vi "Text Description.vi"(11 "Relabel in":refnum<class "AddOuterEnvelope.lvclass">) -> (2 "Description":string, 3 "Relabel out":refnum<class "AddOuterEnvelope.lvclass">)   [LabVIEW 2011, in "Messenging.lvlib" / "AddOuterEnvelope.lvclass"]
uses:
  AddOuterEnvelope.lvclass
  AddOuterEnvelope.lvclass/AddOuterEnvelope.ctl
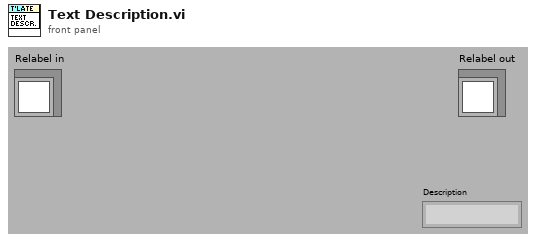
[diagram p1: front panel]
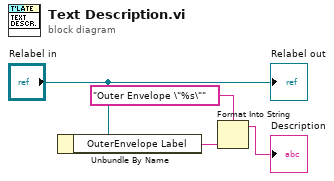
[diagram p0: block diagram]
diagram:
  n1 = Unbundle By Name("Relabel in") -> ("OuterEnvelope Label"=w2:string)
  n2 = Format Into String(format string="Outer Envelope \"%s\"", w2) -> (resulting string=→"Description":string)  [unwired: 2 in, 1 out]
  "Relabel out" <- "Relabel in"
